vi "min.vi"(10 "Numeric":dbl, 11 "Numeric 2":sgl) -> (2 "min":sgl)   [LabVIEW 2022 SP3]
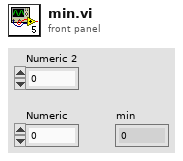
[diagram p1: front panel]
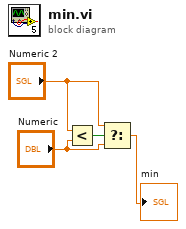
[diagram p0: block diagram]
diagram:
  n1 = Less?(x="Numeric 2", y="Numeric") -> (x < y?=w1:bool)
  n2 = Select(t="Numeric 2", s=w1, f="Numeric") -> (s? t:f=→"min":dbl)
